vi "Ping.vi"(8 "error in (no error)":errorcluster, 9 "timeout in ms (5000)":i32=5000, 11 "Protected Actor Handle in":refnum<class "Protected Actor Handle.lvclass">) -> (0 "error out":errorcluster, 1 "delay in seconds":dbl, 2 "timed out?":bool, 4 "actor quit before receiving ping?":bool)   [LabVIEW 2020, in "Actor Framework.lvlib" / "Protected Actor Handle.lvclass"]
doc: "Sends the Ping Msg to the actor and waits for a reply to know how long the ping took to arrive. Use this VI in a debugger to test whether the actor is still alive."
uses:
  Protected Actor Handle.lvclass
  Ping msg/Ping Msg.lvclass
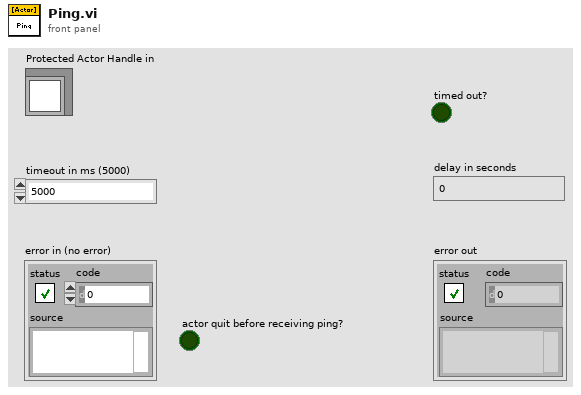
[diagram p1: front panel]
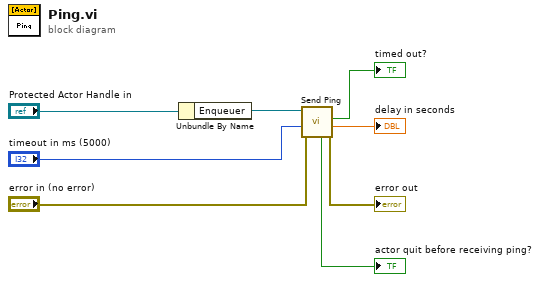
[diagram p0: block diagram]
diagram:
  n1 = Unbundle By Name("Protected Actor Handle in") -> ("Enqueuer"=w7:refnum<class "Message Enqueuer.lvclass">)
  n2 = call "Send Ping.vi"("error in (no error)"="error in (no error)", "timeout in ms (5000)"="timeout in ms (5000)", "Message Enqueuer"=w7) -> ("error out"=→"error out":errorcluster, "delay in seconds"=→"delay in seconds":dbl, "timed out?"=→"timed out?":bool, "actor quit before receiving ping?"=→"actor quit before receiving ping?":bool)  [unwired: 4 in, 1 out]
